vi "TimeInterpDouble_SetMaxTime.vi"(9 "Max Time":dbl, 11 "in TimeInterpDouble":T1) -> (3 "out TimeInterpDouble":T1)   [LabVIEW 2019, in "Trajectory_Library.lvlib"]
doc: "Set the maximum time period that should be stored in the buffer\n\nInputs:\n - In TimeInterpDouble -- Input data cluster.\n - Max Time -- Maximum time period to store in the buffer (seconds)\n\nOutputs:\n - Out TimeInterpDouble -- Updated data cluster."
uses:
  Trajectory_Library.lvlib
  TypeDef/TIME_INTERPOLATABLE_DOUBLE.ctl
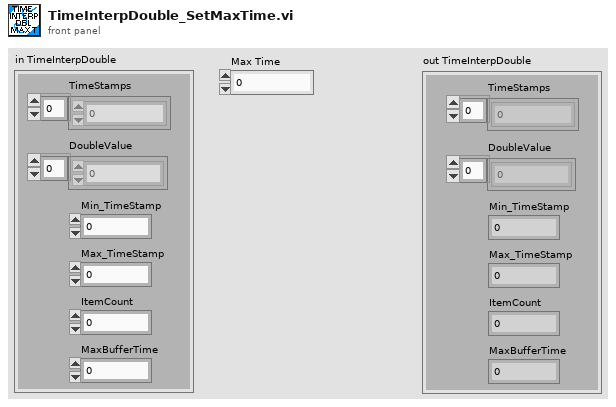
[diagram p1: front panel]
types:
  T1 = typedef "Trajectory_Library.lvlib/TIME_INTERPOLATABLE_DOUBLE.ctl" = cluster{"TimeStamps":dbl[], "DoubleValue":dbl[], "Min_TimeStamp":dbl, "Max_TimeStamp":dbl, "ItemCount":i32, "MaxBufferTime":dbl}
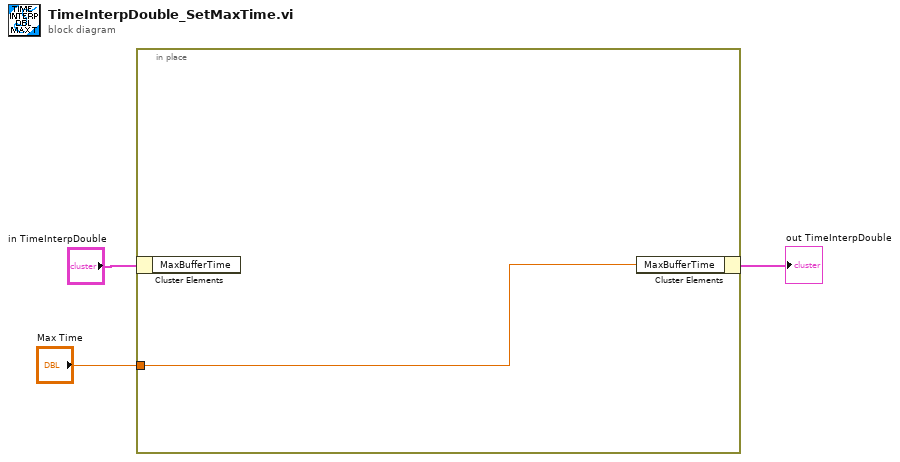
[diagram p0: block diagram]
diagram:
  n1 = in-place {
    in-place-border: "Max Time" -> [w4]
    n2 = in-place-cluster #1("in TimeInterpDouble") -> ()  [unwired: 1 out]
    n3 = in-place-cluster #1("MaxBufferTime"=w4) -> (→"out TimeInterpDouble":T1)
  }
